vi "DumbDash Get Control Type.vi"(10 "reference":refnum<vi>) -> (2 "Type":T1)   [LabVIEW 2015]
uses:
  DumbDash Control Type.ctl
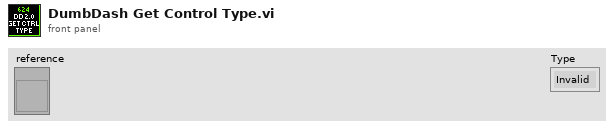
[diagram p1: front panel]
types:
  T1 = typedef "DumbDash Control Type.ctl" = enum16{"Invalid", "Number", "Boolean", "String"}
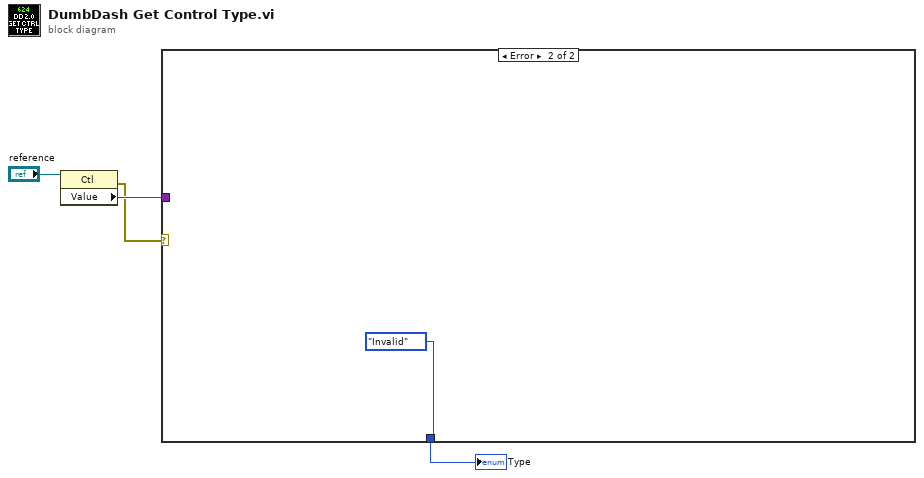
[diagram p0: block diagram]
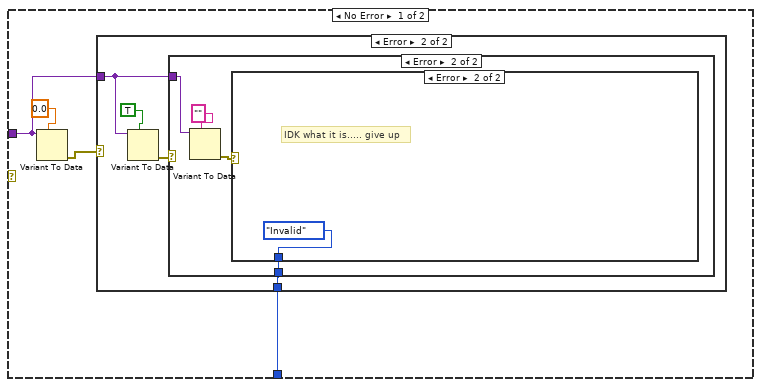
[diagram p2: hidden frame]
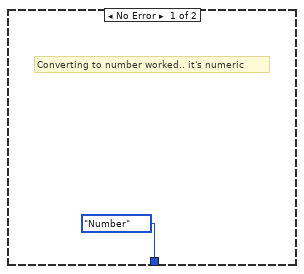
[diagram p3: hidden frame]
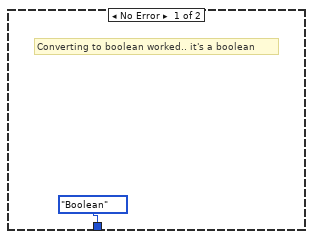
[diagram p4: hidden frame]
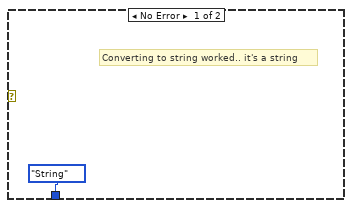
[diagram p5: hidden frame]
diagram:
  n1 = property class="Ctl"(reference="reference") -> (error out=w2:errorcluster, "Value"=w4:variant)  [unwired: 1 in, 1 out]
  n2 = case shown="Error" w2 {
    tunnel: w4 -> [w6 _]
    tunnel: [w5 DumbDash_Control_Type."Invalid"] -> w1
    frame No Error {
      n3 = Variant To Data(type=0.0, Variant=w6) -> (error out=w7:errorcluster)  [unwired: 1 in, 1 out]
      n4 = case shown="Error" w7 {
        tunnel: w6 -> [_ w11]
        tunnel: [DumbDash_Control_Type."Number" w10] -> w5
        frame No Error {
          # "Converting to number worked.. it's numeric"
        }
        frame Error {
          n5 = Variant To Data(type=TRUE, Variant=w11) -> (error out=w12:errorcluster)  [unwired: 1 in, 1 out]
          n6 = case shown="Error" w12 {
            tunnel: w11 -> [_ w18]
            tunnel: [DumbDash_Control_Type."Boolean" w15] -> w10
            frame No Error {
              # "Converting to boolean worked.. it's a boolean"
            }
            frame Error {
              n7 = Variant To Data(type="", Variant=w18) -> (error out=w16:errorcluster)  [unwired: 1 in, 1 out]
              n8 = case shown="Error" w16 {
                tunnel: [DumbDash_Control_Type."String" DumbDash_Control_Type."Invalid"] -> w15
                frame No Error {
                  # "Converting to string worked.. it's a string"
                }
                frame Error {
                  # "IDK what it is..... give up"
                }
              }
            }
          }
        }
      }
    }
    frame Error {
    }
  }
  "Type" <- w1
